vi "EDIT-ME.vi"() -> ()   [LabVIEW 2019]
uses:
  <vilib>/Utility/file.llb/Write Delimited Spreadsheet (string).vi
panel:
  out "Line Clear":dbl
  out "Tank Vent":dbl
  out "String 18":string
  out "String 17":string
  out "String 16":string
  out "String 15":string
  out "String 14":string
  out "String 13":string
  out "String 12":string
  out "String 11":string
  out "String 10":string
  out "String 9":string
  out "String 8":string
  out "String 7":string
  out "String 6":string
  out "String 5":string
  out "String 4":string
  out "String 3":string
  out "String 2":string
  out "String":string
  in  "Logging":bool
  out "Finished 2":bool caption="Complete"
  out "CLOSE VALVES 2":bool caption="Valve Close"
  out "OSV1 Open 2":bool caption="OSV1 Open"
  out "OSV2 Vent 2":bool caption="OSV2 Vent"
  in  "OX Automation 2":bool
  out "Boolean 27":bool
  out "Finished":bool caption="Complete"
  out "CLOSE VALVES":bool caption="Valve Close"
  out "OSV1 Open":bool
  out "OSV2 Vent":bool
  in  "OX Automation":bool
  out "Boolean 23":bool
  out "Valve Close":bool
  out "Automation Complete":bool caption="Complete"
  out "Nitrogen Flow Stop":bool caption="Nitrogen Stop"
  out "OX Flow":bool
  out "Fuel Flow":bool
  out "Ignition":bool
  out "Monitoring":bool caption="Waiting..."
  out "Clear System Delay":dbl
  out "Fire Delay":dbl
  out "Flow Delay":dbl
  in  "OK Button 2":bool
  in  "OK Button":bool
  out "Boolean 28":bool
  out "Ingintor Input":string
  out "Ignition Voltage Signal":dbl format="%#_4g"
  out "Error LC2 2":string
  out "error out  20":errorcluster
  in  "Flow Automation":bool
  out "Boolean 21":bool
  out "Error On Analog 13":string
  out "error out 14":errorcluster
  out "Signal Input Value 3":string
  out "Boolean 26":bool
  in  "OSV5":bool
  out "Boolean 19":bool
  out "Error On Analog 12":string
  out "error out 13":errorcluster
  out "Signal Input Value 2":string
  out "Boolean 25":bool
  in  "OSV4":bool
  out "Boolean 17":bool
  out "Error On Analog 11":string
  out "error out 12":errorcluster
  out "Signal Input Value":string
  out "Boolean 24":bool
  out "Boolean 15":bool
  out "Error On Analog 10":string
  out "error out 11":errorcluster
  out "Signal Input Value":string
  out "Boolean 13":bool
  out "Error On Analog 9":string
  out "error out 10":errorcluster
  out "Signal Input Value":string
  out "Boolean 11":bool
  out "Error On Analog 8":string
  out "error out 9":errorcluster
  out "Signal Input Value":string
  out "Boolean 7":bool
  out "Error On Analog 7":string
  out "error out 8":errorcluster
  out "Signal Input Value":string
  in  "OSV3":bool
  out "Boolean 22":bool
  in  "OSV2":bool
  out "Boolean 20":bool
  in  "OSV1":bool
  out "Boolean 18":bool
  in  "FSV5":bool
  out "Boolean 16":bool
  in  "FSV4":bool
  out "Boolean 14":bool
  in  "FSV3":bool
  out "Boolean 12":bool
  in  "FSV2":bool
  out "Boolean 10":bool
  in  "FSV1":bool
  out "Boolean 6":bool
  out "Boolean 4":bool
  out "Boolean":bool
  out "LC2":dbl format="%#_4g"
  out "Error LC2":string
  out "error out  19":errorcluster
  out "LC1":dbl format="%#_4g"
  out "Error LC1":string
  out "error out  18":errorcluster
  out "CPS0":dbl format="%#_4g"
  out "Error CPS0":string
  out "error out  17":errorcluster
  out "CTS0":dbl format="%#_4g"
  out "Error CTS0":string
  out "error out  16":errorcluster
  out "OTS3":dbl format="%#_4g"
  out "Error OTS3":string
  out "error out  15":errorcluster
  out "OTS2":dbl format="%#_4g"
  out "Error OTS2":string
  out "error out  14":errorcluster
  out "OTS1":dbl format="%#_4g"
  out "Error OTS1":string
  out "error out  13":errorcluster
  out "OPS5":dbl format="%#_4g"
  out "Error OPS5":string
  out "error out  12":errorcluster
  out "OPS4":dbl format="%#_4g"
  out "Error OPS4":string
  out "error out  11":errorcluster
  out "OPS3":dbl format="%#_4g"
  out "Error OPS3":string
  out "error out  10":errorcluster
  out "OPS2":dbl format="%#_4g"
  out "Error OPS2":string
  out "error out  9":errorcluster
  out "OPS1":dbl format="%#_4g"
  out "FTS1 2":dbl format="%#_4g"
  out "Error FTS2":string
  out "error out  7":errorcluster
  out "FTS1":dbl format="%#_4g"
  out "FPS4":dbl format="%#_4g"
  out "FPS3":dbl format="%#_4g"
  out "FPS2":dbl format="%#_4g"
  out "FPS1":dbl format="%#_4g"
  out "Error OPS1":string
  out "error out  8":errorcluster
  out "Samples":i32
  out "Boolean 9":bool
  out "Error FTS1":string
  out "error out  6":errorcluster
  out "Error FPS4":string
  out "error out  5":errorcluster
  out "Error FPS3":string
  out "error out  4":errorcluster
  out "Error On Analog 6":string
  out "error out 7":errorcluster
  out "Signal Input Value":string
  out "Error On SV2":string
  out "error out 6":errorcluster
  out "Signal Input Value":string
  out "Error On SV1":string
  out "error out 5":errorcluster
  out "Signal Input Value":string
  out "error out  3":errorcluster
  out "Error FPS1":string
  out "ConnectionType Out":i32
  out "DeviceType Out":i32
  in  "Identifier":string="LJM_idANY"
  in  "ConnectionType":string="LJM_ctANY"
  in  "DeviceType":string="LJM_dtANY"
  out "Error  On System":string
  out "error out":errorcluster
  in  "stop":bool
  out "error out  2":errorcluster
  out "Error  FPS2":string
  in  "DATA DOWNLOAD FILE PATH":path
  # "SOAR BASE 11 Hot Fire Test DAQ and Controls"
  # "DATA FLOW CONTROL"
  # "FSV1 (NC)"
  # "FSV2 (NC)"
  # "FSV3 (NC)"
  # "FSV4 (NC)"
  # "FSV5 (NO)"
  # "Labjack Device Controls/Parameters"
  # "OSV1 (NC)"
  # "OSV2 (NC)"
  # "OSV3 (NC)"
  # "OSV4 (NC)"
  # "OSV5 (NO)"
  # "Data Download & Logging"
  # "MASTER FLOW"
  # "Ignition Monitoring For Flow Automation"
  # "OX Vent Automation"
  # "FLOW AUTOMATION"
  # "Fuel Vent Automation"
  # "Fuel Vent Automation Sequence"
  # "OX Vent Automation Sequence"
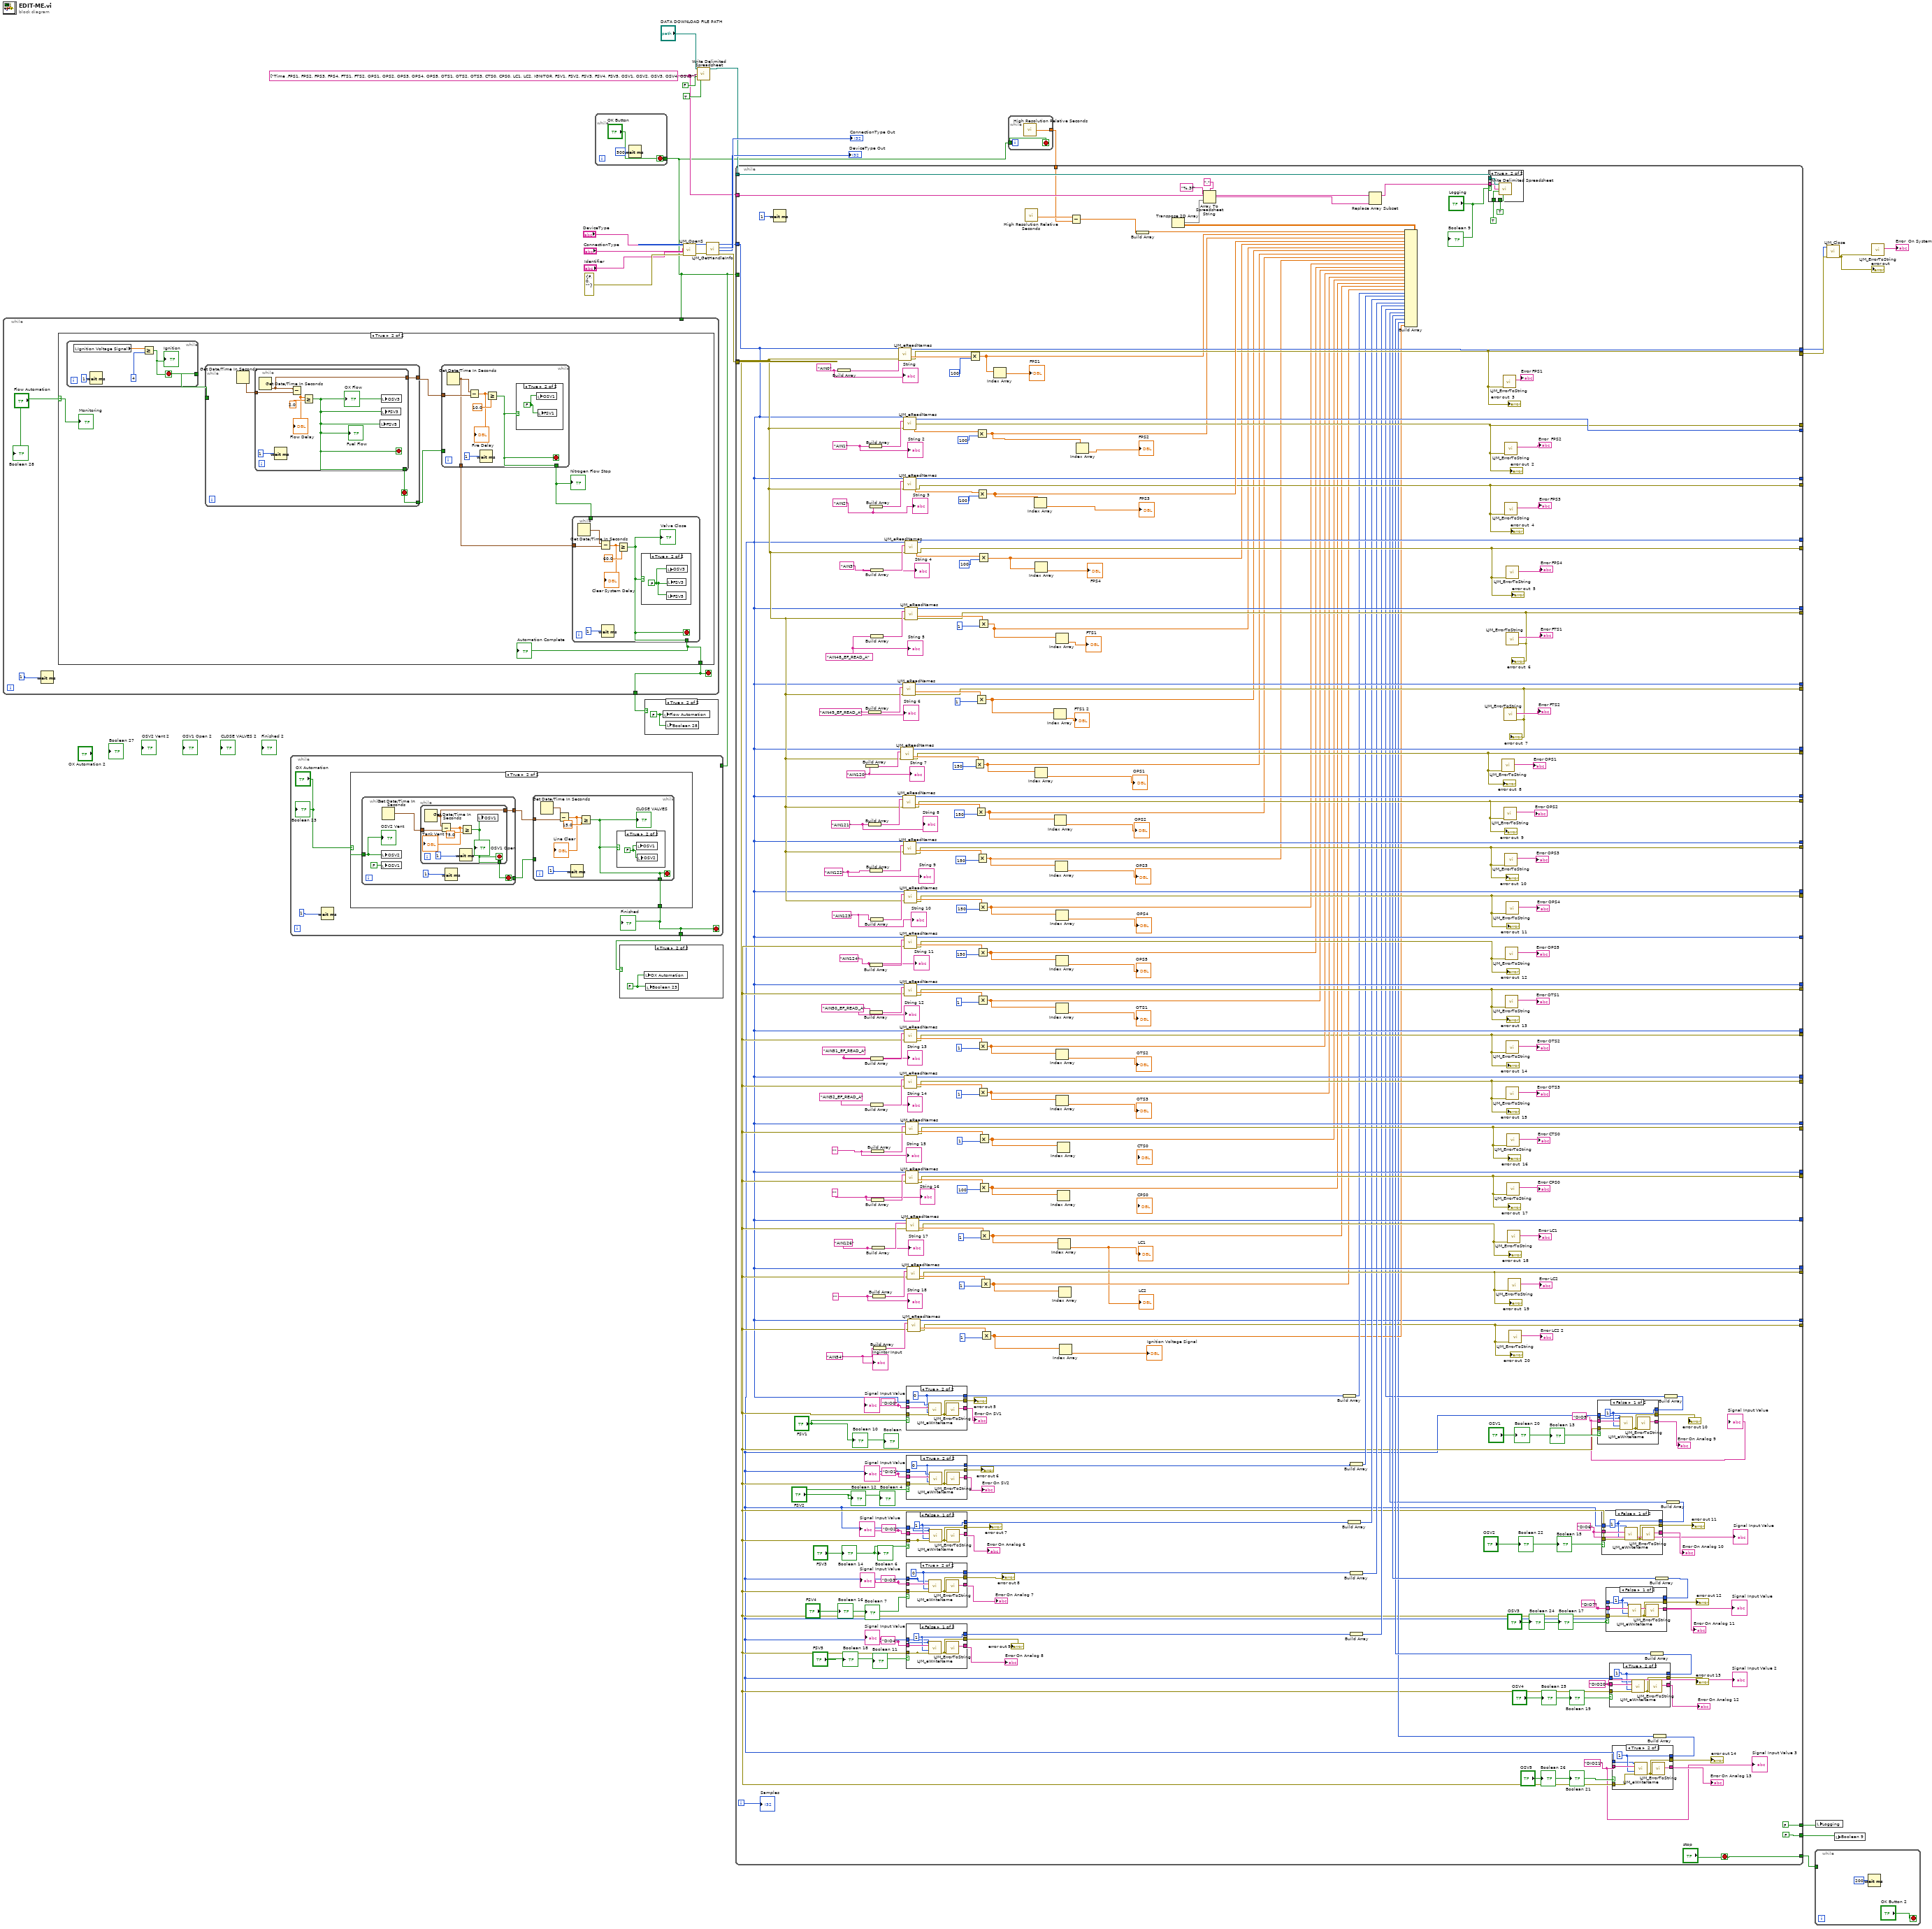
[diagram p0: block diagram]
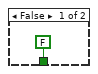
[diagram p3: hidden frame]
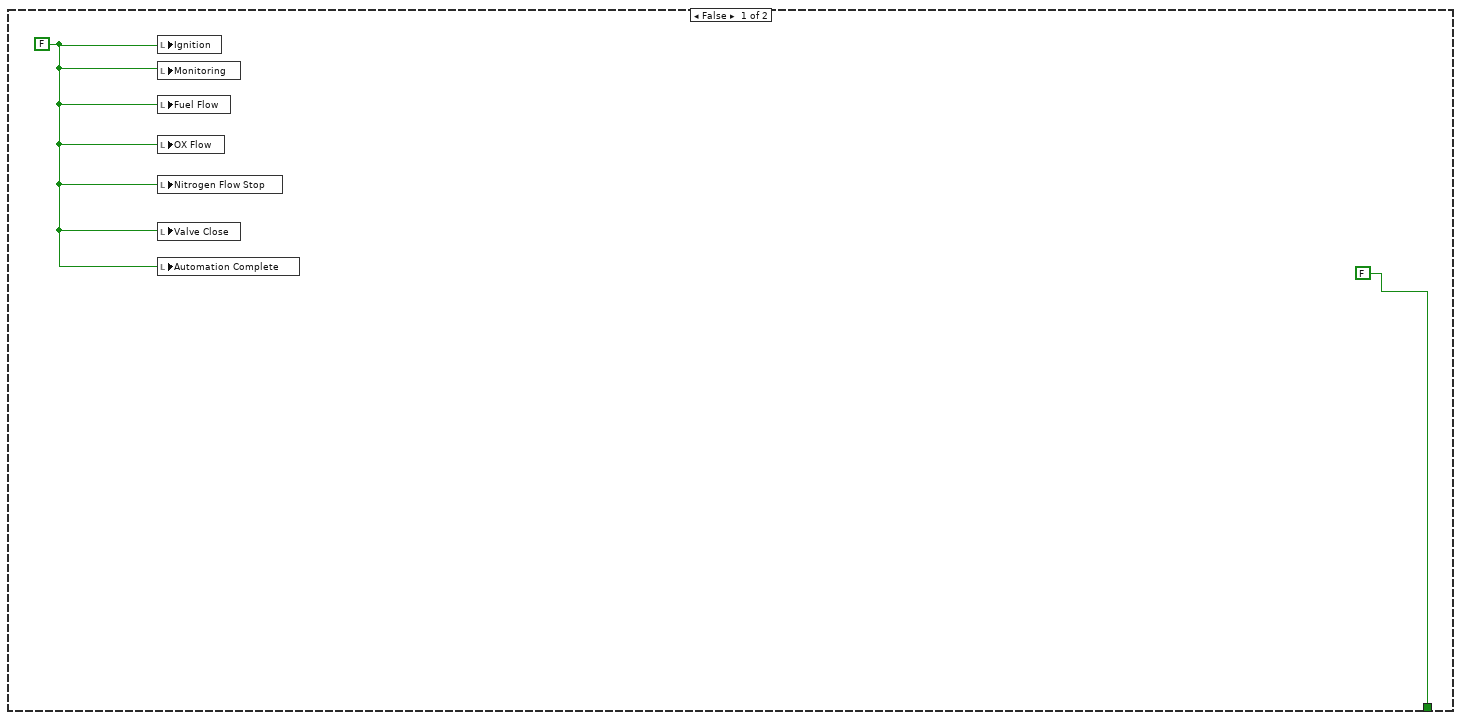
[diagram p6: hidden frame]
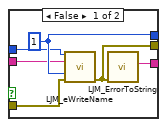
[diagram p9: hidden frame]
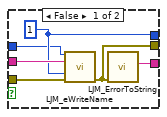
[diagram p10: hidden frame]
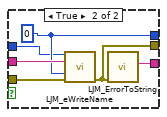
[diagram p11: hidden frame]
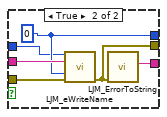
[diagram p12: hidden frame]
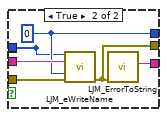
[diagram p13: hidden frame]
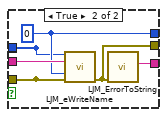
[diagram p14: hidden frame]
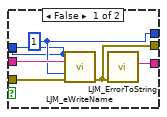
[diagram p15: hidden frame]
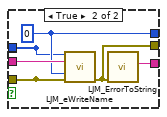
[diagram p16: hidden frame]
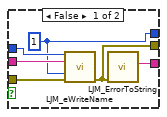
[diagram p17: hidden frame]
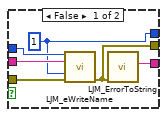
[diagram p18: hidden frame]
diagram:
  w15 = string[] ["Time ,FPS1, FPS2, FPS3, FPS4, FTS1, FTS2, OPS1, OPS2, OPS3, OPS4, OPS5, OTS1, OTS2, OTS3, CTS0, CPS0, LC1, LC2, IGNITOR, FSV1, FSV2, FSV3, FSV4, FSV5, OSV1, OSV2, OSV3, OSV4, OSV5"]
  n1 = while {
    tunnel: ["OK Button"] -> w2
    stop <- "OK Button" stop-if-true
    n2 = Wait (ms)(milliseconds to wait=u32 500) -> ()  [unwired: 1 out]
  }
  n3 = while {
    tunnel: [w29] -> w5
    tunnel: w2 -> [_]
    stop <- w29 stop-if-true
    n4 = Wait (ms)(milliseconds to wait=u32 1) -> ()  [unwired: 1 out]
    n5 = case shown="True" "Flow Automation" {
      selector: "Flow Automation" -> [_ w37]
      tunnel: [FALSE w36] -> w29
      frame False {
        w32 = FALSE
        n6 = local write "Ignition"(w32) -> ()
        n7 = local write "Monitoring"(w32) -> ()
        n8 = local write "Fuel Flow"(w32) -> ()
        n9 = local write "OX Flow"(w32) -> ()
        n10 = local write "Nitrogen Flow Stop"(w32) -> ()
        n11 = local write "Valve Close"(w32) -> ()
        n12 = local write "Automation Complete"(w32) -> ()
      }
      frame True {
        n13 = while {
          tunnel: [w65] -> w39
          stop <- w65 stop-if-true
          n14 = local read "Ignition Voltage Signal"() -> (w64:dbl)
          n15 = Wait (ms)(milliseconds to wait=u32 1) -> ()  [unwired: 1 out]
          n16 = Greater Or Equal?(x=w64, y=4) -> (x >= y?=w65:bool)
          "Ignition" <- w65
        }
        n17 = while {
          tunnel: w39 -> [_]
          tunnel: [w56] -> w38
          tunnel: [w55] -> w40
          stop <- w56 stop-if-true
          n18 = Get Date/Time In Seconds() -> (seconds since 1Jan1904=w57:timestamp)
          n19 = while {
            tunnel: w57 -> [w61]
            tunnel: [w58] -> w56
            tunnel: [w59] -> w55
            stop <- w58 stop-if-true
            n20 = Get Date/Time In Seconds() -> (seconds since 1Jan1904=w59:timestamp)
            n21 = Wait (ms)(milliseconds to wait=u32 1) -> ()  [unwired: 1 out]
            n22 = Subtract(x=w59, y=w61) -> (x-y=w60:dbl)
            "Flow Delay" <- w60
            n23 = Greater Or Equal?(x=w60, y=2.0) -> (x >= y?=w58:bool)
            "OX Flow" <- w58
            "Fuel Flow" <- w58
            n24 = local write "FSV5"(w58) -> ()
            n25 = local write "OSV3"(w58) -> ()
            n26 = local write "FSV3"(w58) -> ()
          }
        }
        n27 = while {
          tunnel: [w50] -> w35
          tunnel: w40 -> [w51]
          tunnel: w38 -> [_]
          tunnel: [w48] -> w34
          stop <- w50 stop-if-true
          n28 = Get Date/Time In Seconds() -> (seconds since 1Jan1904=w48:timestamp)
          n29 = Subtract(x=w48, y=w51) -> (x-y=w52:dbl)
          "Fire Delay" <- w52
          n30 = Wait (ms)(milliseconds to wait=u32 1) -> ()  [unwired: 1 out]
          n31 = Greater Or Equal?(x=w52, y=10.0) -> (x >= y?=w50:bool)
          n32 = case shown="True" w50 {
            frame False {
            }
            frame True {
              w54 = FALSE
              n33 = local write "OSV1"(w54) -> ()
              n34 = local write "FSV1"(w54) -> ()
            }
          }
        }
        "Nitrogen Flow Stop" <- w35
        n35 = while {
          tunnel: [w42] -> w36
          tunnel: w34 -> [w45]
          tunnel: w35 -> [_]
          stop <- w42 stop-if-true
          n36 = Get Date/Time In Seconds() -> (seconds since 1Jan1904=w46:timestamp)
          n37 = Subtract(x=w46, y=w45) -> (x-y=w43:dbl)
          "Clear System Delay" <- w43
          n38 = Wait (ms)(milliseconds to wait=u32 1) -> ()  [unwired: 1 out]
          n39 = Greater Or Equal?(x=w43, y=60.0) -> (x >= y?=w42:bool)
          "Valve Close" <- w42
          n40 = case shown="True" w42 {
            frame False {
            }
            frame True {
              w47 = FALSE
              n41 = local write "OSV3"(w47) -> ()
              n42 = local write "FSV5"(w47) -> ()
              n43 = local write "FSV3"(w47) -> ()
            }
          }
        }
        "Automation Complete" <- w36
        "Monitoring" <- w37
      }
    }
    "Boolean 28" <- "Flow Automation"
  }
  n44 = while {
    tunnel: w2 -> [_]
    tunnel: [w69] -> w1
    stop <- w69 stop-if-true
    n45 = Wait (ms)(milliseconds to wait=u32 1) -> ()  [unwired: 1 out]
    n46 = case shown="True" "OX Automation" {
      selector: "OX Automation" -> [_ w75]
      tunnel: [FALSE w72] -> w69
      frame False {
      }
      frame True {
        n47 = while {
          tunnel: w75 -> [w88]
          tunnel: [w85] -> w74
          tunnel: [w84] -> w73
          stop <- w85 stop-if-true
          n48 = local write "OSV2"(w88) -> ()
          n49 = local write "OSV1"(FALSE) -> ()
          n50 = Get Date/Time In Seconds() -> (seconds since 1Jan1904=w86:timestamp)
          n51 = while {
            tunnel: w86 -> [w94]
            tunnel: [w92] -> w85
            tunnel: [w91] -> w84
            stop <- w92 stop-if-true
            n52 = Get Date/Time In Seconds() -> (seconds since 1Jan1904=w91:timestamp)
            n53 = Subtract(x=w91, y=w94) -> (x-y=w89:dbl)
            "Tank Vent" <- w89
            n54 = Wait (ms)(milliseconds to wait=u32 1) -> ()  [unwired: 1 out]
            n55 = Greater Or Equal?(x=w89, y=75.0) -> (x >= y?=w92:bool)
            "OSV1 Open" <- w92
            n56 = local write "OSV1"(w92) -> ()
          }
          n57 = Wait (ms)(milliseconds to wait=u32 1) -> ()  [unwired: 1 out]
          "OSV2 Vent" <- w88
        }
        n58 = while {
          tunnel: w74 -> [_]
          tunnel: w73 -> [w80]
          tunnel: [w78] -> w72
          stop <- w78 stop-if-true
          n59 = Get Date/Time In Seconds() -> (seconds since 1Jan1904=w81:timestamp)
          n60 = Subtract(x=w81, y=w80) -> (x-y=w76:dbl)
          "Line Clear" <- w76
          n61 = Wait (ms)(milliseconds to wait=u32 1) -> ()  [unwired: 1 out]
          n62 = Greater Or Equal?(x=w76, y=15.0) -> (x >= y?=w78:bool)
          "CLOSE VALVES" <- w78
          n63 = case shown="True" w78 {
            frame False {
            }
            frame True {
              w82 = FALSE
              n64 = local write "OSV1"(w82) -> ()
              n65 = local write "OSV2"(w82) -> ()
            }
          }
        }
      }
    }
    "Finished" <- w69
    "Boolean 23" <- "OX Automation"
  }
  n66 = case shown="True" w1 {
    frame False {
    }
    frame True {
      w95 = FALSE
      n67 = local write "OX Automation"(w95) -> ()
      n68 = local write "Boolean 23"(w95) -> ()
    }
  }
  n69 = case shown="True" w5 {
    frame False {
    }
    frame True {
      w96 = FALSE
      n70 = local write "Flow Automation"(w96) -> ()
      n71 = local write "Boolean 28"(w96) -> ()
    }
  }
  n72 = call "LJM_OpenS.vi"("error in"=errorcluster {"status"=FALSE, "code"=0, "source"=""} ("error in (no error)"), "Identifier"="Identifier", "ConnectionType"="ConnectionType", "DeviceType"="DeviceType") -> ("error out"=w24:errorcluster, "Handle"=w23:i32)  [unwired: 6 in]
  n73 = call-poly <vilib>:"Write Delimited Spreadsheet.vi"("file path (dialog if empty)"="DATA DOWNLOAD FILE PATH", "1D data"=w15, "append to file? (new file:F)"=FALSE, "transpose? (no:F)"=TRUE) -> ("new file path (Not A Path if cancelled)"=w10:path)  [unwired: 10 in, 1 out]
  n74 = call "LJM_GetHandleInfo.vi"("error in"=w24, "Handle In"=w23) -> ("error out"=w7:errorcluster, "ConnectionType"=→"DeviceType Out":i32, "DeviceType"=→"ConnectionType Out":i32, "Handle Out"=w6:i32)  [unwired: 2 in, 4 out]
  n75 = while {
    tunnel: w2 -> [w98]
    tunnel: [w97] -> w3
    stop <- w98 stop-if-true
    n76 = call <vilib>:"High Resolution Relative Seconds.vi"() -> ("relative seconds"=w97:dbl)
  }
  n77 = while {
    tunnel: w7 -> [w140]
    tunnel: w7 -> [_]
    tunnel: w15 -> [w327]
    tunnel: [w322] -> w13
    tunnel: [w321] -> w12
    tunnel: [w320] -> _
    tunnel: [w319] -> _
    tunnel: [w318] -> _
    tunnel: [w317] -> _
    tunnel: [w316] -> _
    tunnel: [w315] -> _
    tunnel: [w314] -> _
    tunnel: [w313] -> _
    tunnel: w10 -> [w312]
    tunnel: [FALSE] -> w4
    tunnel: [FALSE] -> w9
    tunnel: [w300] -> _
    tunnel: [w299] -> _
    tunnel: [w284] -> _
    tunnel: [w283] -> _
    tunnel: [w274] -> _
    tunnel: [w273] -> _
    tunnel: [w266] -> _
    tunnel: [w265] -> _
    tunnel: [w258] -> _
    tunnel: [w257] -> _
    tunnel: [w249] -> _
    tunnel: [w242] -> _
    tunnel: [w241] -> _
    tunnel: [w234] -> _
    tunnel: [w198] -> _
    tunnel: [w227] -> _
    tunnel: [w226] -> _
    tunnel: [w221] -> _
    tunnel: [w220] -> _
    tunnel: [w214] -> _
    tunnel: [w213] -> _
    tunnel: [w206] -> _
    tunnel: [w200] -> _
    tunnel: [w199] -> _
    tunnel: [w184] -> _
    tunnel: [w183] -> _
    tunnel: w2 -> [_]
    tunnel: ["stop"] -> w8
    tunnel: w6 -> [w136]
    tunnel: w3 -> [w102]
    i -> [w308]
    stop <- "stop" stop-if-true
    w101 = "AIN54"
    w117 = ""
    w118 = "AIN126"
    w119 = ""
    w120 = ""
    w122 = "AIN52_EF_READ_A"
    w123 = "AIN51_EF_READ_A"
    w124 = "AIN50_EF_READ_A"
    w125 = "AIN124"
    w126 = "AIN123"
    w127 = "AIN122"
    w128 = "AIN121"
    w129 = "AIN120"
    w130 = "AIN49_EF_READ_A"
    w131 = "AIN48_EF_READ_A"
    w132 = "AIN3"
    w133 = "AIN2"
    w134 = "AIN1"
    w135 = "AIN0"
    w108 = "DIO21"
    w109 = "DIO20"
    w110 = "DIO7"
    w111 = "DIO6"
    w104 = "DIO5"
    w112 = "DIO4"
    w113 = "DIO3"
    w114 = "DIO2"
    w115 = "DIO1"
    w116 = "DIO0"
    n78 = Wait (ms)(milliseconds to wait=u32 1 ("millisecond timer value")) -> ()  [unwired: 1 out]
    n79 = Build Array(w135) -> (w137:string[])
    n80 = Build Array(w129) -> (w304:string[])
    n81 = Build Array(w128) -> (w279:string[])
    n82 = Build Array(w130) -> (w289:string[])
    n83 = Build Array(w134) -> (w348:string[])
    n84 = Build Array(w133) -> (w343:string[])
    n85 = Build Array(w127) -> (w271:string[])
    n86 = Build Array(w125) -> (w255:string[])
    n87 = Build Array(w124) -> (w247:string[])
    n88 = Build Array(w126) -> (w263:string[])
    n89 = Build Array(w123) -> (w239:string[])
    n90 = Build Array(w122) -> (w232:string[])
    n91 = Build Array(w132) -> (w340:string[])
    n92 = Build Array(w131) -> (w337:string[])
    n93 = Build Array(w120) -> (w121:string[])
    n94 = Build Array(w119) -> (w218:string[])
    n95 = Build Array(w118) -> (w211:string[])
    n96 = Build Array(w117) -> (w204:string[])
    n97 = Build Array(w101) -> (w189:string[])
    n98 = call "LJM_eReadNames.vi"("Handle In"=w136, "aNames"=w137, "error in"=w140) -> ("Handle Out"=w321:i32, "aValuesOut"=w334:dbl[], "error out"=w322:errorcluster)  [unwired: 9 in, 1 out]
    "error out  3" <- w322
    n99 = call "LJM_eReadNames.vi"("Handle In"=w136, "aNames"=w304, "error in"=w140) -> ("Handle Out"=w300:i32, "aValuesOut"=w301:dbl[], "error out"=w299:errorcluster)  [unwired: 9 in, 1 out]
    "error out  8" <- w299
    n100 = call "LJM_eReadNames.vi"("Handle In"=w136, "aNames"=w279, "error in"=w140) -> ("Handle Out"=w274:i32, "aValuesOut"=w276:dbl[], "error out"=w273:errorcluster)  [unwired: 9 in, 1 out]
    "error out  9" <- w273
    n101 = call "LJM_eReadNames.vi"("Handle In"=w136, "aNames"=w289, "error in"=w140) -> ("Handle Out"=w284:i32, "aValuesOut"=w286:dbl[], "error out"=w283:errorcluster)  [unwired: 9 in, 1 out]
    "error out  7" <- w283
    n102 = call "LJM_eReadNames.vi"("Handle In"=w136, "aNames"=w348, "error in"=w140) -> ("Handle Out"=w320:i32, "aValuesOut"=w333:dbl[], "error out"=w319:errorcluster)  [unwired: 9 in, 1 out]
    "error out  2" <- w319
    n103 = call "LJM_eReadNames.vi"("Handle In"=w136, "aNames"=w343, "error in"=w140) -> ("Handle Out"=w317:i32, "aValuesOut"=w331:dbl[], "error out"=w318:errorcluster)  [unwired: 9 in, 1 out]
    "error out  4" <- w318
    n104 = call "LJM_eReadNames.vi"("Handle In"=w136, "aNames"=w271, "error in"=w140) -> ("Handle Out"=w266:i32, "aValuesOut"=w268:dbl[], "error out"=w265:errorcluster)  [unwired: 9 in, 1 out]
    "error out  10" <- w265
    n105 = call "LJM_eReadNames.vi"("Handle In"=w136, "aNames"=w255, "error in"=w140) -> ("Handle Out"=w249:i32, "aValuesOut"=w252:dbl[], "error out"=w250:errorcluster)  [unwired: 9 in, 1 out]
    "error out  12" <- w250
    n106 = call "LJM_eReadNames.vi"("Handle In"=w136, "aNames"=w247, "error in"=w140) -> ("Handle Out"=w242:i32, "aValuesOut"=w244:dbl[], "error out"=w241:errorcluster)  [unwired: 9 in, 1 out]
    "error out  13" <- w241
    n107 = call "LJM_eReadNames.vi"("Handle In"=w136, "aNames"=w263, "error in"=w140) -> ("Handle Out"=w258:i32, "aValuesOut"=w260:dbl[], "error out"=w257:errorcluster)  [unwired: 9 in, 1 out]
    "error out  11" <- w257
    n108 = call "LJM_eReadNames.vi"("Handle In"=w136, "aNames"=w239, "error in"=w140) -> ("Handle Out"=w234:i32, "aValuesOut"=w236:dbl[], "error out"=w198:errorcluster)  [unwired: 9 in, 1 out]
    "error out  14" <- w198
    n109 = call "LJM_eReadNames.vi"("Handle In"=w136, "aNames"=w232, "error in"=w140) -> ("Handle Out"=w227:i32, "aValuesOut"=w229:dbl[], "error out"=w226:errorcluster)  [unwired: 9 in, 1 out]
    "error out  15" <- w226
    n110 = call "LJM_eReadNames.vi"("Handle In"=w136, "aNames"=w340, "error in"=w140) -> ("Handle Out"=w315:i32, "aValuesOut"=w329:dbl[], "error out"=w316:errorcluster)  [unwired: 9 in, 1 out]
    "error out  5" <- w316
    n111 = call "LJM_eReadNames.vi"("Handle In"=w136, "aNames"=w337, "error in"=w140) -> ("Handle Out"=w313:i32, "aValuesOut"=w330:dbl[], "error out"=w314:errorcluster)  [unwired: 9 in, 1 out]
    "error out  6" <- w314
    n112 = call "LJM_eReadNames.vi"("Handle In"=w136, "aNames"=w121, "error in"=w140) -> ("Handle Out"=w221:i32, "aValuesOut"=w222:dbl[], "error out"=w220:errorcluster)  [unwired: 9 in, 1 out]
    "error out  16" <- w220
    n113 = call "LJM_eReadNames.vi"("Handle In"=w136, "aNames"=w218, "error in"=w140) -> ("Handle Out"=w214:i32, "aValuesOut"=w215:dbl[], "error out"=w213:errorcluster)  [unwired: 9 in, 1 out]
    "error out  17" <- w213
    n114 = call "LJM_eReadNames.vi"("Handle In"=w136, "aNames"=w211, "error in"=w140) -> ("Handle Out"=w206:i32, "aValuesOut"=w208:dbl[], "error out"=w207:errorcluster)  [unwired: 9 in, 1 out]
    "error out  18" <- w207
    n115 = case shown="True" "FSV1" {
      tunnel: w136 -> [w460 w464]
      tunnel: w116 -> [w461 w468]
      tunnel: w140 -> [w462 w465]
      tunnel: [w459 w467] -> w181
      tunnel: [w458 w466] -> w180
      tunnel: [w457 w463] -> w178
      frame False {
        w457 = 1
        n116 = call "LJM_eWriteName.vi"("Handle In"=w460, "Name"=w461, "Value"=w457, "error in"=w462) -> ("error out"=w459:errorcluster)  [unwired: 10 in, 1 out]
        n117 = call "LJM_ErrorToString.vi"("error in"=w459) -> ("String"=w458:string)  [unwired: 10 in]
      }
      frame True {
        w463 = 0
        n118 = call "LJM_eWriteName.vi"("Handle In"=w464, "Name"=w468, "Value"=w463, "error in"=w465) -> ("error out"=w467:errorcluster)  [unwired: 10 in, 1 out]
        n119 = call "LJM_ErrorToString.vi"("error in"=w467) -> ("String"=w466:string)  [unwired: 10 in]
      }
    }
    "error out 5" <- w181
    "Error On SV1" <- w180
    n120 = case shown="True" "FSV4" {
      tunnel: w136 -> [w421 w428]
      tunnel: w113 -> [w426 w432]
      tunnel: [w425 w431] -> w168
      tunnel: [w424 w430] -> w167
      tunnel: [w423 w429] -> w169
      tunnel: [w421 w428] -> _
      tunnel: w140 -> [w422 w427]
      frame False {
        w423 = 1
        n121 = call "LJM_eWriteName.vi"("Handle In"=w421, "Name"=w426, "Value"=w423, "error in"=w422) -> ("error out"=w425:errorcluster)  [unwired: 10 in, 1 out]
        n122 = call "LJM_ErrorToString.vi"("error in"=w425) -> ("String"=w424:string)  [unwired: 10 in]
      }
      frame True {
        w429 = 0
        n123 = call "LJM_eWriteName.vi"("Handle In"=w428, "Name"=w432, "Value"=w429, "error in"=w427) -> ("error out"=w431:errorcluster)  [unwired: 10 in, 1 out]
        n124 = call "LJM_ErrorToString.vi"("error in"=w431) -> ("String"=w430:string)  [unwired: 10 in]
      }
    }
    "error out 8" <- w168
    "Error On Analog 7" <- w167
    n125 = case shown="False" "FSV5" {
      tunnel: [w410 w416] -> _
      tunnel: w112 -> [w414 w420]
      tunnel: [w413 w419] -> w163
      tunnel: [w412 w418] -> w164
      tunnel: [w411 w417] -> w165
      tunnel: w136 -> [w410 w416]
      tunnel: [w409 w415] -> _
      tunnel: w140 -> [w409 w415]
      frame False {
        w411 = 1
        n126 = call "LJM_eWriteName.vi"("Handle In"=w410, "Name"=w414, "Value"=w411, "error in"=w409) -> ("error out"=w413:errorcluster)  [unwired: 10 in, 1 out]
        n127 = call "LJM_ErrorToString.vi"("error in"=w413) -> ("String"=w412:string)  [unwired: 10 in]
      }
      frame True {
        w417 = 0
        n128 = call "LJM_eWriteName.vi"("Handle In"=w416, "Name"=w420, "Value"=w417, "error in"=w415) -> ("error out"=w419:errorcluster)  [unwired: 10 in, 1 out]
        n129 = call "LJM_ErrorToString.vi"("error in"=w419) -> ("String"=w418:string)  [unwired: 10 in]
      }
    }
    "error out 9" <- w163
    "Error On Analog 8" <- w164
    n130 = case shown="True" "FSV2" {
      tunnel: w136 -> [w449 w453]
      tunnel: w115 -> [w450 w456]
      tunnel: [w448 w455] -> w176
      tunnel: [w447 w454] -> w177
      tunnel: [w446 w452] -> w175
      tunnel: w140 -> [w445 w451]
      frame False {
        w446 = 1
        n131 = call "LJM_eWriteName.vi"("Handle In"=w449, "Name"=w450, "Value"=w446, "error in"=w445) -> ("error out"=w448:errorcluster)  [unwired: 10 in, 1 out]
        n132 = call "LJM_ErrorToString.vi"("error in"=w448) -> ("String"=w447:string)  [unwired: 10 in]
      }
      frame True {
        w452 = 0
        n133 = call "LJM_eWriteName.vi"("Handle In"=w453, "Name"=w456, "Value"=w452, "error in"=w451) -> ("error out"=w455:errorcluster)  [unwired: 10 in, 1 out]
        n134 = call "LJM_ErrorToString.vi"("error in"=w455) -> ("String"=w454:string)  [unwired: 10 in]
      }
    }
    "error out 6" <- w176
    "Error On SV2" <- w177
    n135 = case shown="False" "FSV3" {
      tunnel: [w433 w439] -> _
      tunnel: w114 -> [w438 w444]
      tunnel: [w437 w443] -> w171
      tunnel: [w436 w442] -> w172
      tunnel: [w435 w441] -> w173
      tunnel: [w434 w440] -> _
      tunnel: w140 -> [w434 w440]
      tunnel: w136 -> [w433 w439]
      frame False {
        w435 = 1
        n136 = call "LJM_eWriteName.vi"("Handle In"=w433, "Name"=w438, "Value"=w435, "error in"=w434) -> ("error out"=w437:errorcluster)  [unwired: 10 in, 1 out]
        n137 = call "LJM_ErrorToString.vi"("error in"=w437) -> ("String"=w436:string)  [unwired: 10 in]
      }
      frame True {
        w441 = 0
        n138 = call "LJM_eWriteName.vi"("Handle In"=w439, "Name"=w444, "Value"=w441, "error in"=w440) -> ("error out"=w443:errorcluster)  [unwired: 10 in, 1 out]
        n139 = call "LJM_ErrorToString.vi"("error in"=w443) -> ("String"=w442:string)  [unwired: 10 in]
      }
    }
    "error out 7" <- w171
    "Error On Analog 6" <- w172
    n140 = call "LJM_eReadNames.vi"("Handle In"=w136, "aNames"=w204, "error in"=w140) -> ("Handle Out"=w200:i32, "aValuesOut"=w201:dbl[], "error out"=w199:errorcluster)  [unwired: 9 in, 1 out]
    "error out  19" <- w199
    n141 = call "LJM_eReadNames.vi"("Handle In"=w136, "aNames"=w189, "error in"=w140) -> ("Handle Out"=w184:i32, "aValuesOut"=w186:dbl[], "error out"=w183:errorcluster)  [unwired: 9 in, 1 out]
    "error out  20" <- w183
    n142 = Multiply(x=w334, y=100) -> (x*y=w298:dbl[])
    n143 = Multiply(x=w301, y=150) -> (x*y=w280:dbl[])
    n144 = Multiply(x=w276, y=150) -> (x*y=w272:dbl[])
    n145 = Multiply(x=w286, y=1) -> (x*y=w282:dbl[])
    n146 = Multiply(x=w333, y=100) -> (x*y=w296:dbl[])
    n147 = Multiply(x=w331, y=100) -> (x*y=w332:dbl[])
    n148 = Multiply(x=w268, y=150) -> (x*y=w264:dbl[])
    n149 = Multiply(x=w252, y=150) -> (x*y=w248:dbl[])
    n150 = Multiply(x=w244, y=1) -> (x*y=w240:dbl[])
    n151 = Multiply(x=w260, y=150) -> (x*y=w256:dbl[])
    n152 = Multiply(x=w236, y=1) -> (x*y=w233:dbl[])
    n153 = Multiply(x=w229, y=1) -> (x*y=w225:dbl[])
    n154 = Multiply(x=w329, y=100) -> (x*y=w292:dbl[])
    n155 = Multiply(x=w330, y=1) -> (x*y=w291:dbl[])
    n156 = Multiply(x=w222, y=1) -> (x*y=w219:dbl[])
    n157 = Multiply(x=w215, y=100) -> (x*y=w212:dbl[])
    n158 = Multiply(x=w208, y=1) -> (x*y=w205:dbl[])
    n159 = Multiply(x=w201, y=1) -> (x*y=w197:dbl[])
    n160 = Multiply(x=w186, y=1) -> (x*y=w185:dbl[])
    n161 = Index Array(array=w298) -> (element=→"FPS1":dbl)  [unwired: 1 in]
    n162 = call <vilib>:"High Resolution Relative Seconds.vi"() -> ("relative seconds"=w106:dbl)
    n163 = Index Array(array=w332) -> (element=→"FPS3":dbl)  [unwired: 1 in]
    n164 = Index Array(array=w280) -> (element=→"OPS1":dbl)  [unwired: 1 in]
    n165 = Index Array(array=w292) -> (element=→"FPS4":dbl)  [unwired: 1 in]
    n166 = Index Array(array=w282) -> (element=→"FTS1 2":dbl)  [unwired: 1 in]
    n167 = Index Array(array=w272) -> (element=→"OPS2":dbl)  [unwired: 1 in]
    n168 = Index Array(array=w264) -> (element=→"OPS3":dbl)  [unwired: 1 in]
    n169 = Index Array(array=w291) -> (element=→"FTS1":dbl)  [unwired: 1 in]
    n170 = Index Array(array=w248) -> (element=→"OPS5":dbl)  [unwired: 1 in]
    n171 = Index Array(array=w240) -> (element=→"OTS1":dbl)  [unwired: 1 in]
    n172 = Index Array(array=w256) -> (element=→"OPS4":dbl)  [unwired: 1 in]
    n173 = Index Array(array=w233) -> (element=→"OTS2":dbl)  [unwired: 1 in]
    n174 = Index Array(array=w225) -> (element=→"OTS3":dbl)  [unwired: 1 in]
    n175 = Index Array(array=w219) -> ()  [unwired: 1 in, 1 out]
    n176 = Index Array(array=w212) -> ()  [unwired: 1 in, 1 out]
    n177 = Index Array(array=w205) -> (element=→"LC1" →"LC2":dbl)  [unwired: 1 in]
    n178 = Index Array(array=w197) -> ()  [unwired: 1 in, 1 out]
    n179 = Index Array(array=w185) -> (element=→"Ignition Voltage Signal":dbl)  [unwired: 1 in]
    n180 = Subtract(x=w106, y=w102) -> (x-y=w105:dbl)
    n181 = Index Array(array=w296) -> (element=→"FPS2":dbl)  [unwired: 1 in]
    n182 = Build Array(w105) -> (w305:dbl[])
    n183 = Build Array(w178) -> (w196:i32[])
    n184 = Build Array(w173) -> (w194:i32[])
    n185 = Build Array(w175) -> (w195:i32[])
    n186 = Build Array(w169) -> (w193:i32[])
    n187 = Build Array(w165) -> (w192:i32[])
    n188 = call "LJM_ErrorToString.vi"("error in"=w299) -> ("String"=→"Error OPS1":string)  [unwired: 10 in]
    n189 = call "LJM_ErrorToString.vi"("error in"=w322) -> ("String"=→"Error FPS1":string)  [unwired: 10 in]
    n190 = call "LJM_ErrorToString.vi"("error in"=w273) -> ("String"=→"Error OPS2":string)  [unwired: 10 in]
    n191 = call "LJM_ErrorToString.vi"("error in"=w283) -> ("String"=→"Error FTS2":string)  [unwired: 10 in]
    n192 = call "LJM_ErrorToString.vi"("error in"=w319) -> ("String"=→"Error  FPS2":string)  [unwired: 10 in]
    n193 = call "LJM_ErrorToString.vi"("error in"=w318) -> ("String"=→"Error FPS3":string)  [unwired: 10 in]
    n194 = call "LJM_ErrorToString.vi"("error in"=w265) -> ("String"=→"Error OPS3":string)  [unwired: 10 in]
    n195 = call "LJM_ErrorToString.vi"("error in"=w250) -> ("String"=→"Error OPS5":string)  [unwired: 10 in]
    n196 = call "LJM_ErrorToString.vi"("error in"=w241) -> ("String"=→"Error OTS1":string)  [unwired: 10 in]
    n197 = call "LJM_ErrorToString.vi"("error in"=w257) -> ("String"=→"Error OPS4":string)  [unwired: 10 in]
    n198 = call "LJM_ErrorToString.vi"("error in"=w198) -> ("String"=→"Error OTS2":string)  [unwired: 10 in]
    n199 = call "LJM_ErrorToString.vi"("error in"=w226) -> ("String"=→"Error OTS3":string)  [unwired: 10 in]
    n200 = call "LJM_ErrorToString.vi"("error in"=w316) -> ("String"=→"Error FPS4":string)  [unwired: 10 in]
    n201 = call "LJM_ErrorToString.vi"("error in"=w314) -> ("String"=→"Error FTS1":string)  [unwired: 10 in]
    n202 = call "LJM_ErrorToString.vi"("error in"=w220) -> ("String"=→"Error CTS0":string)  [unwired: 10 in]
    n203 = call "LJM_ErrorToString.vi"("error in"=w213) -> ("String"=→"Error CPS0":string)  [unwired: 10 in]
    n204 = call "LJM_ErrorToString.vi"("error in"=w207) -> ("String"=→"Error LC1":string)  [unwired: 10 in]
    n205 = call "LJM_ErrorToString.vi"("error in"=w199) -> ("String"=→"Error LC2":string)  [unwired: 10 in]
    n206 = call "LJM_ErrorToString.vi"("error in"=w183) -> ("String"=→"Error LC2 2":string)  [unwired: 10 in]
    n207 = case shown="False" "OSV1" {
      tunnel: [w398 w404] -> _
      tunnel: w104 -> [w402 w408]
      tunnel: [w401 w407] -> w158
      tunnel: [w400 w406] -> w159
      tunnel: [w399 w405] -> w160
      tunnel: w136 -> [w398 w404]
      tunnel: w140 -> [w397 w403]
      frame False {
        w399 = 1
        n208 = call "LJM_eWriteName.vi"("Handle In"=w398, "Name"=w402, "Value"=w399, "error in"=w397) -> ("error out"=w401:errorcluster)  [unwired: 10 in, 1 out]
        n209 = call "LJM_ErrorToString.vi"("error in"=w401) -> ("String"=w400:string)  [unwired: 10 in]
      }
      frame True {
        w405 = 0
        n210 = call "LJM_eWriteName.vi"("Handle In"=w404, "Name"=w408, "Value"=w405, "error in"=w403) -> ("error out"=w407:errorcluster)  [unwired: 10 in, 1 out]
        n211 = call "LJM_ErrorToString.vi"("error in"=w407) -> ("String"=w406:string)  [unwired: 10 in]
      }
    }
    "error out 10" <- w158
    "Error On Analog 9" <- w159
    n212 = case shown="False" "OSV2" {
      tunnel: w111 -> [w390 w396]
      tunnel: [w389 w395] -> w153
      tunnel: [w388 w394] -> w154
      tunnel: w140 -> [w385 w393]
      tunnel: [w387 w392] -> w156
      tunnel: w136 -> [w386 w391]
      frame False {
        w387 = 1
        n213 = call "LJM_eWriteName.vi"("Handle In"=w386, "Name"=w390, "Value"=w387, "error in"=w385) -> ("error out"=w389:errorcluster)  [unwired: 10 in, 1 out]
        n214 = call "LJM_ErrorToString.vi"("error in"=w389) -> ("String"=w388:string)  [unwired: 10 in]
      }
      frame True {
        w392 = 0
        n215 = call "LJM_eWriteName.vi"("Handle In"=w391, "Name"=w396, "Value"=w392, "error in"=w393) -> ("error out"=w395:errorcluster)  [unwired: 10 in, 1 out]
        n216 = call "LJM_ErrorToString.vi"("error in"=w395) -> ("String"=w394:string)  [unwired: 10 in]
      }
    }
    "error out 11" <- w153
    "Error On Analog 10" <- w154
    n217 = case shown="False" "OSV3" {
      tunnel: w110 -> [w378 w384]
      tunnel: [w377 w383] -> w149
      tunnel: [w376 w382] -> w150
      tunnel: w140 -> [w374 w381]
      tunnel: [w375 w380] -> w152
      tunnel: w136 -> [w373 w379]
      frame False {
        w375 = 1
        n218 = call "LJM_eWriteName.vi"("Handle In"=w373, "Name"=w378, "Value"=w375, "error in"=w374) -> ("error out"=w377:errorcluster)  [unwired: 10 in, 1 out]
        n219 = call "LJM_ErrorToString.vi"("error in"=w377) -> ("String"=w376:string)  [unwired: 10 in]
      }
      frame True {
        w380 = 0
        n220 = call "LJM_eWriteName.vi"("Handle In"=w379, "Name"=w384, "Value"=w380, "error in"=w381) -> ("error out"=w383:errorcluster)  [unwired: 10 in, 1 out]
        n221 = call "LJM_ErrorToString.vi"("error in"=w383) -> ("String"=w382:string)  [unwired: 10 in]
      }
    }
    "error out 12" <- w149
    "Error On Analog 11" <- w150
    n222 = case shown="True" "OSV4" {
      tunnel: w109 -> [w366 w372]
      tunnel: [w365 w371] -> w146
      tunnel: [w364 w370] -> w147
      tunnel: w140 -> [w362 w369]
      tunnel: [w363 w368] -> w148
      tunnel: w136 -> [w361 w367]
      frame False {
        w363 = 1
        n223 = call "LJM_eWriteName.vi"("Handle In"=w361, "Name"=w366, "Value"=w363, "error in"=w362) -> ("error out"=w365:errorcluster)  [unwired: 10 in, 1 out]
        n224 = call "LJM_ErrorToString.vi"("error in"=w365) -> ("String"=w364:string)  [unwired: 10 in]
      }
      frame True {
        w368 = 1
        n225 = call "LJM_eWriteName.vi"("Handle In"=w367, "Name"=w372, "Value"=w368, "error in"=w369) -> ("error out"=w371:errorcluster)  [unwired: 10 in, 1 out]
        n226 = call "LJM_ErrorToString.vi"("error in"=w371) -> ("String"=w370:string)  [unwired: 10 in]
      }
    }
    "error out 13" <- w146
    "Error On Analog 12" <- w147
    n227 = case shown="True" "OSV5" {
      tunnel: [w354 w360] -> w142
      tunnel: [w353 w359] -> w141
      tunnel: w140 -> [w349 w358]
      tunnel: [w352 w356] -> w145
      tunnel: w136 -> [w351 w355]
      tunnel: w108 -> [w350 w357]
      frame False {
        w352 = 1
        n228 = call "LJM_eWriteName.vi"("Handle In"=w351, "Name"=w350, "Value"=w352, "error in"=w349) -> ("error out"=w354:errorcluster)  [unwired: 10 in, 1 out]
        n229 = call "LJM_ErrorToString.vi"("error in"=w354) -> ("String"=w353:string)  [unwired: 10 in]
      }
      frame True {
        w356 = 1
        n230 = call "LJM_eWriteName.vi"("Handle In"=w355, "Name"=w357, "Value"=w356, "error in"=w358) -> ("error out"=w360:errorcluster)  [unwired: 10 in, 1 out]
        n231 = call "LJM_ErrorToString.vi"("error in"=w360) -> ("String"=w359:string)  [unwired: 10 in]
      }
    }
    "error out 14" <- w142
    "Error On Analog 13" <- w141
    n232 = Build Array(w148) -> (w190:i32[])
    n233 = Build Array(w145) -> (w143:i32[])
    n234 = Build Array(w152) -> (w191:i32[])
    n235 = Build Array(w160) -> (w161:i32[])
    n236 = Build Array(w156) -> (w157:i32[])
    n237 = Build Array(w305, w298, w296, w332, w292, w291, w282, w280, w272, w264, w256, w248, w240, w233, w225, w219, w212, w205, w197, w196, w195, w194, w193, w192, w161, w157, w191, w190, w143, w185) -> (w324:dbl[][])
    n238 = Transpose 2D Array(2D array=w324) -> (transposed array=w323:dbl[][])
    n239 = Array To Spreadsheet String(delimiter (Tab)=",", array=w323, 3:"%.3f") -> (spreadsheet string=w328:string)
    n240 = Replace Array Subset "Replace Array Subset"(array=w327, new element=w328) -> (w311:string[])  [unwired: 1 in]
    n241 = case shown="True" "Logging" {
      tunnel: w312 -> [_ w472]
      tunnel: w311 -> [_ w471]
      tunnel: TRUE -> [_ w470]
      tunnel: TRUE -> [_ w469]
      frame False {
      }
      frame True {
        n242 = call-poly <vilib>:"Write Delimited Spreadsheet.vi"("file path (dialog if empty)"=w472, "1D data"=w471, "append to file? (new file:F)"=w470, "transpose? (no:F)"=w469) -> ()  [unwired: 10 in, 2 out]
      }
    }
    "Signal Input Value" <- w116
    "Signal Input Value" <- w115
    "Signal Input Value" <- w114
    "Boolean 9" <- "Logging"
    "Samples" <- w308
    "Boolean 16" <- "FSV4"
    "Boolean 18" <- "FSV5"
    "Boolean 20" <- "OSV1"
    "Boolean 22" <- "OSV2"
    "Boolean 10" <- "FSV1"
    "Boolean" <- "FSV1"
    "Boolean 4" <- "FSV2"
    "Boolean 12" <- "FSV2"
    "Boolean 14" <- "FSV3"
    "Boolean 6" <- "FSV3"
    "Signal Input Value" <- w113
    "Boolean 7" <- "FSV4"
    "Signal Input Value" <- w112
    "Boolean 11" <- "FSV5"
    "Signal Input Value" <- w104
    "Boolean 13" <- "OSV1"
    "Signal Input Value" <- w111
    "Boolean 15" <- "OSV2"
    "Boolean 24" <- "OSV3"
    "Signal Input Value" <- w110
    "Boolean 17" <- "OSV3"
    "Boolean 25" <- "OSV4"
    "Signal Input Value 2" <- w109
    "Boolean 19" <- "OSV4"
    "Boolean 26" <- "OSV5"
    "Signal Input Value 3" <- w108
    "Boolean 21" <- "OSV5"
    "Ingintor Input" <- w101
    "String" <- w135
    "String 2" <- w134
    "String 3" <- w133
    "String 4" <- w132
    "String 5" <- w131
    "String 6" <- w130
    "String 7" <- w129
    "String 8" <- w128
    "String 9" <- w127
    "String 10" <- w126
    "String 11" <- w125
    "String 12" <- w124
    "String 13" <- w123
    "String 14" <- w122
    "String 15" <- w120
    "String 16" <- w119
    "String 17" <- w118
    "String 18" <- w117
  }
  n243 = while {
    tunnel: w8 -> [_]
    stop <- "OK Button 2" stop-if-true
    n244 = Wait (ms)(milliseconds to wait=u32 200) -> ()  [unwired: 1 out]
  }
  n245 = local write "Logging"(w4) -> ()
  n246 = call "LJM_Close.vi"("error in"=w13, "Handle"=w12) -> ("error out"=w11:errorcluster)  [unwired: 9 in]
  "error out" <- w11
  n247 = local write "Boolean 9"(w9) -> ()
  n248 = call "LJM_ErrorToString.vi"("error in"=w11) -> ("String"=→"Error  On System":string)  [unwired: 10 in]
